vi "Create File.vi"(8 "error in (no error)":errorcluster, 11 "TIFF in":refnum<class "TIFF.lvclass">) -> (0 "error out":errorcluster, 3 "TIFF out":refnum<class "TIFF.lvclass">)   [LabVIEW 2018, in "BinaryTIFF.lvlib" / "TIFF.lvclass"]
uses:
  TIFF.lvclass
  TIFF.lvclass/TIFF.ctl
  <vilib>/Utility/error.llb/Error Cluster From Error Code.vi
  <vilib>/ErrorRing/Error Ring.xnode
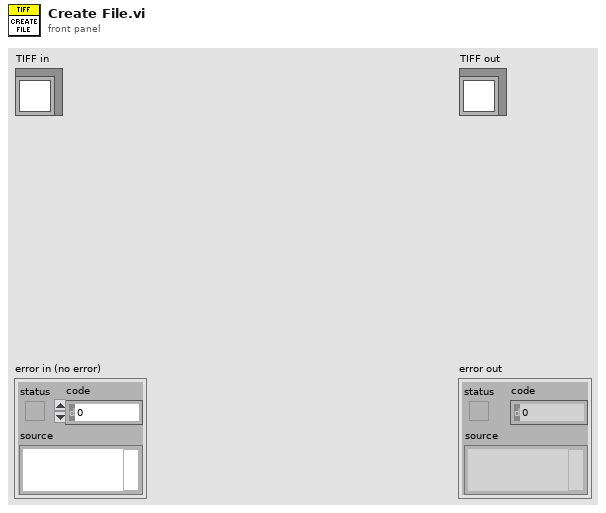
[diagram p1: front panel]
types:
  T1 = enum16{"open", "replace", "create", "open or create", "replace or create", "replace or create with confirmation"}
  T2 = enum16{"<not opened>", "Open for Read", "Open for Write"}
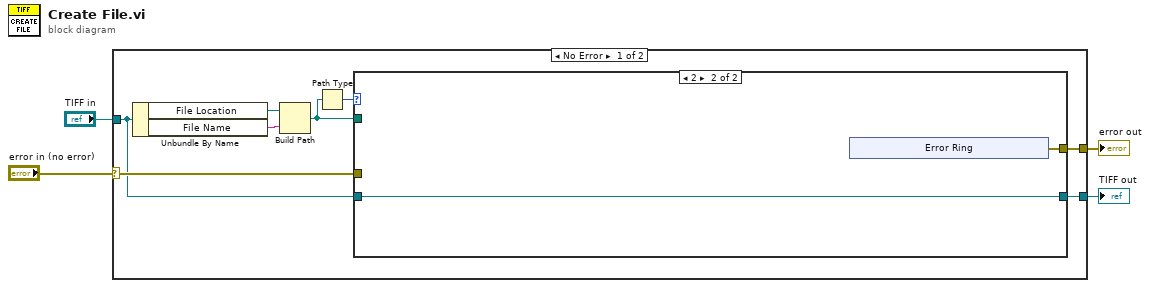
[diagram p0: block diagram]
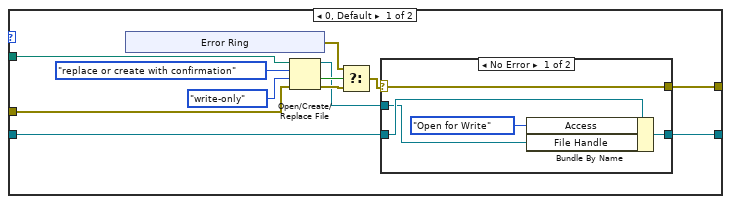
[diagram p2: hidden frame]
diagram:
  n1 = case shown="No Error" "error in (no error)" {
    selector: "error in (no error)" -> [w9 w43]
    tunnel: [w5 w43] -> w3
    tunnel: [w6 w42] -> w1
    tunnel: "TIFF in" -> [w7 w42]
    frame No Error {
      n2 = Unbundle By Name(w7) -> ("File Location"=w12:path, "File Name"=w11:string)
      n3 = Build Path(base path=w12, name or relative path=w11) -> (appended path=w8:path)
      n4 = Path Type(1:w8) -> (0:w10:i16)
      n5 = case shown="2" w10 {
        tunnel: w9 -> [w22 _]
        tunnel: [w14 w36] -> w5
        tunnel: w8 -> [w21 _]
        tunnel: w7 -> [w20 w37]
        tunnel: [w19 w37] -> w6
        frame 0, Default {
          n6 = xnode "Error Ring"() -> ("error out"=w13:errorcluster)
          n7 = Open/Create/Replace File(file path (use dialog)=w21, error in=w22, operation (0:open)=T1."replace or create with confirmation", access (0:read/write)=enum16{"read/write", "read-only", "write-only"}."write-only") -> (refnum out=w15:refnum<file>, cancelled=w18:bool, error out=w17:errorcluster)  [unwired: 2 in]
          n8 = Select(t=w13, s=w18, f=w17) -> (s? t:f=w16:errorcluster)
          n9 = case shown="No Error" w16 {
            selector: w16 -> [w29 w34]
            tunnel: w20 -> [w33 w35]
            tunnel: [w32 w35] -> w19
            tunnel: w15 -> [w30 _]
            tunnel: [w29 w34] -> w14
            frame No Error {
              n10 = Bundle By Name(cluster=w33, "Access"=T2."Open for Write" ("File Info.Access"), "File Handle"=w30) -> (w32:refnum<class "TIFF.lvclass">)
            }
            frame Error {
            }
          }
        }
        frame 2 {
          n11 = xnode "Error Ring"() -> ("error out"=w36:errorcluster)
        }
      }
    }
    frame Error {
    }
  }
  "error out" <- w3
  "TIFF out" <- w1
